vi "Make All Variables Temporary.vi"(11 "connection ID":refnum<k5>) -> (3 "connection ID 2":refnum<k5>)   [LabVIEW 2017]
doc: "This VI will be called when a connection fails and the client or server is becoming isolated. All variable names and values are retained, but the IDs may not be the same when it rejoins with a server. So the variables IDs are freed and converted to negative (temporary) ID values."
uses:
  <vilib>/Rock Robotics/Network Tables/Make Table Operation.ctl
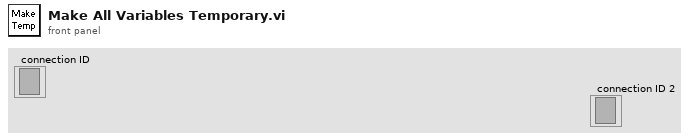
[diagram p1: front panel]
types:
  T1 = enum16{"Update Field", "Read Field", "Assign Field"}
  T2 = typedef "Make Table Operation.ctl" = enum16{"Get or Add Field", "Get Field or Add Temp", "Replace Temp ID", "Get Field ID - No Add", "Get Table Field IDs", "Get Field ID Info", "Move Field to Temp", "Validate", "Remove Field", "Remove All"}
  T3 = typedef "Field ID.ctl" = i32
  T4 = typedef "Field Data.ctl" = cluster{"Dbl":dbl, "String":string, "Type":T5, "Boolean":bool, "Sequence #":T6, "Flags":u8}
  T5 = typedef "Field Type.ctl" = enum8{"Invalid", "Bool", "Numeric", "String", "Raw", "Boolean Array", "Numeric Array", "String Array", "RPC"}
  T6 = typedef "Sequence.ctl" = u16
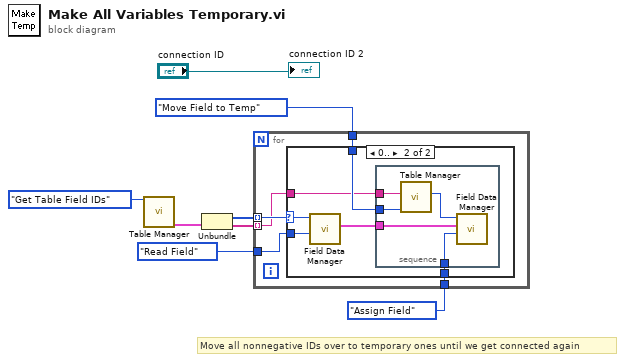
[diagram p0: block diagram]
diagram:
  # "Move all nonnegative IDs over to temporary ones until we get connected again"
  n1 = call <vilib>:"Table Manager.vi"("Operation"=Make_Table_Operation."Get Table Field IDs") -> ("Entries"=w6:cluster{"Entry IDs":T3[], "Names":string[]})  [unwired: 7 in, 3 out]
  n2 = Unbundle(w6) -> ("Entry IDs"=w7:T3[], "Names"=w1:string[])
  n3 = for {
    tunnel: w7 -> [w13] mode=indexing
    tunnel: Make_Table_Operation."Move Field to Temp" ("Operation") -> [w12]
    tunnel: T1."Read Field" ("Operation") -> [w11]
    tunnel: T1."Assign Field" ("Operation") -> [w10]
    tunnel: w1 -> [w9] mode=indexing
    n4 = case shown="0.." w13 {
      selector: w13 -> [_ w19]
      tunnel: w12 -> [_ w17]
      tunnel: w11 -> [_ w16]
      tunnel: w10 -> [_ w15]
      tunnel: w9 -> [_ w14]
      frame Default {
      }
      frame 0.. {
        n5 = call <vilib>:"Field Data Manager.vi"("Operation"=w16, "Field ID"=w19) -> ("Field Value Out"=w18:T4)  [unwired: 8 in, 1 out]
        n6 = stacked-sequence {
          tunnel: w18 -> [w23]
          tunnel: w17 -> [w22]
          tunnel: w15 -> [w21]
          tunnel: w14 -> [w20]
          frame #0 {
            n7 = call <vilib>:"Table Manager.vi"("Operation"=w22, "Entry Name"=w20) -> ("Entry ID"=w24:T3)  [unwired: 6 in, 3 out]
            n8 = call <vilib>:"Field Data Manager.vi"("Operation"=w21, "Field Value In"=w23, "Field ID"=w24) -> ()  [unwired: 7 in, 2 out]
          }
        }
      }
    }
  }
  "connection ID 2" <- "connection ID"
